vi "Load Settings from XML.vi"(8 "error in (no error)":errorcluster, 11 "Settings in":T1) -> (0 "error out":errorcluster, 3 "Settings out":T1)   [LabVIEW 2022 SP3, in "pm Settings.lvlib"]
doc: "Attempts to load previous user specified settings from an XML file.\n\nThis VI will not generate an error. If a suitable XML file can't be loaded and parsed then it will simply return the default settings."
uses:
  pm Settings.lvlib
  Settings.ctl
  Acquisition/Hardware Configuration.ctl
  Acquisition/Signal Type.ctl
  Logging/Logging Configuration.ctl
  <vilib>/Utility/xml.llb/Read From XML File(string).vi
  <vilib>/Utility/xml.llb/Write to XML File(string).vi
  Acquisition/pm Acquisition.lvlib
  Logging/pm Logging.lvlib
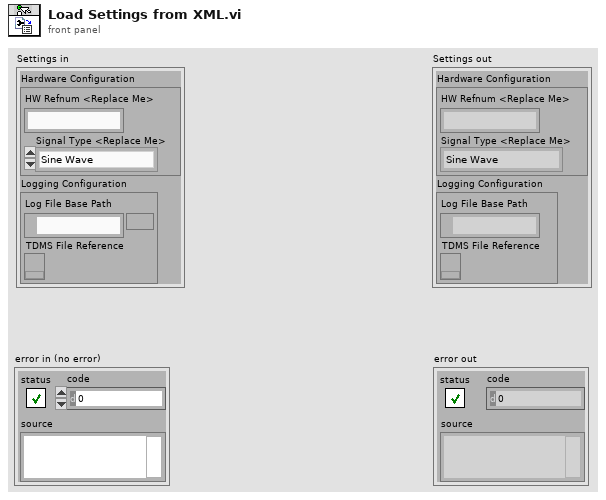
[diagram p1: front panel]
types:
  T1 = typedef "pm Settings.lvlib/Settings.ctl" = cluster{"Hardware Configuration":T2, "Logging Configuration":T4}
  T2 = typedef "pm Acquisition.lvlib/Hardware Configuration.ctl" = cluster{"HW Refnum <Replace Me>":string, "Signal Type <Replace Me>":T3}
  T3 = typedef "pm Acquisition.lvlib/Signal Type.ctl" = enum16{"Sine Wave", "Square with Noise"}
  T4 = typedef "pm Logging.lvlib/Logging Configuration.ctl" = cluster{"Log File Base Path":path, "TDMS File Reference":refnum<k34>}
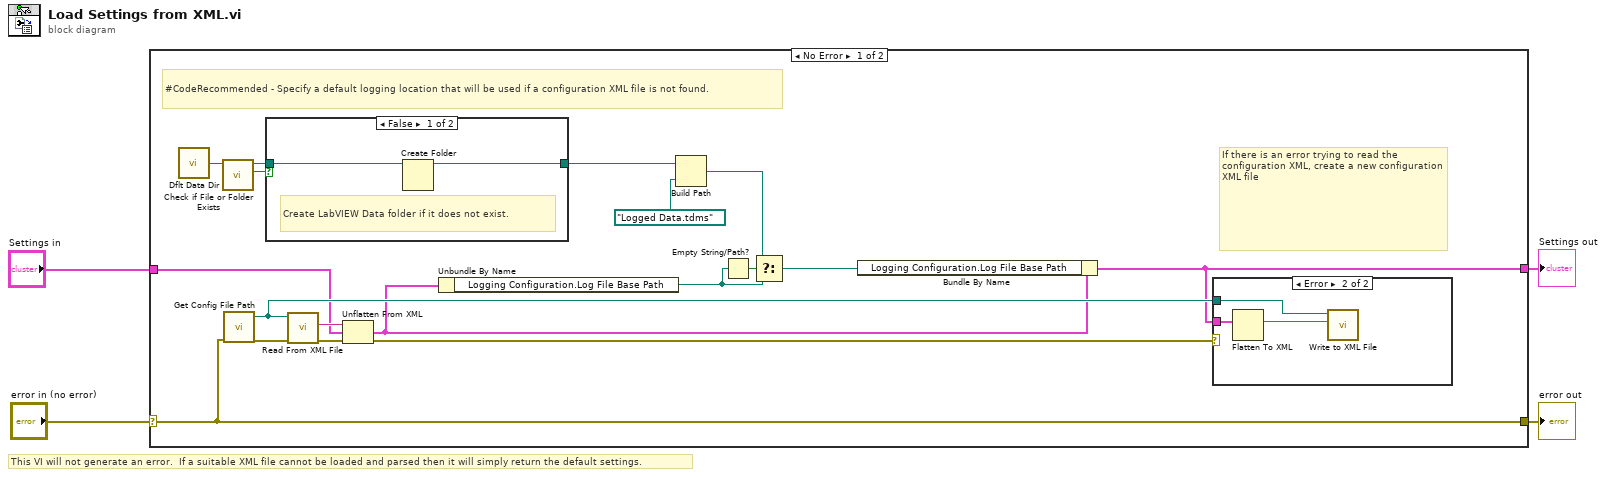
[diagram p0: block diagram]
diagram:
  # "This VI will not generate an error.  If a suitable XML file cannot be loaded and parsed then it will simply return the default settings."
  n1 = case shown="No Error" "error in (no error)" {
    selector: "error in (no error)" -> [w20 w30]
    tunnel: [w20 w30] -> w3
    tunnel: "Settings in" -> [w15 w29]
    tunnel: [w9 w29] -> w1
    frame No Error {
      # "If there is an error trying to read the configuration XML, create a new configuration XML file"
      # "#CodeRecommended - Specify a default logging location that will be used if a configuration XML file is not found."
      n2 = call <vilib>:"Dflt Data Dir.vi"() -> ("App:Default Data Directory"=w8:path)
      n3 = call <vilib>:"Check if File or Folder Exists.vi"("path"=w8) -> ("file or folder exists?"=w7:bool, "dup path"=w6:path)  [unwired: 8 in, 1 out]
      n4 = call "Get Config File Path.vi"("error in (no error)"=w20) -> ("error out"=w22:errorcluster, "XML File Path"=w18:path)  [unwired: 9 in]
      n5 = case shown="False" w7 {
        tunnel: w6 -> [w24 w25]
        tunnel: [w23 w25] -> w5
        frame False {
          # "Create LabVIEW Data folder if it does not exist."
          n6 = Create Folder(path (use dialog)=w24) -> (created path=w23:path)  [unwired: 2 in, 2 out]
        }
        frame True {
        }
      }
      n7 = call-poly <vilib>:"Read From XML File.vi"("error in (no error)"=w22, "XML File Path"=w18) -> ("error out"=w17:errorcluster, "XML Elements"=w21:string)  [unwired: 7 in, 1 out]
      n8 = Unflatten From XML(xml string=w21, type=w15, error in (no error)=w17) -> (value=w11:T1, error out=w16:errorcluster)
      n9 = Unbundle By Name(w11) -> ("Logging Configuration.Log File Base Path"=w13:path)
      n10 = Build Path(base path=w5, name or relative path=path "Logged Data.tdms" ("App:Default Data Directory")) -> (appended path=w12:path)
      n11 = Empty String/Path?(string/path=w13) -> (empty?=w14:bool)
      n12 = Select(t=w12, s=w14, f=w13) -> (s? t:f=w10:path)
      n13 = Bundle By Name(cluster=w11, "Logging Configuration.Log File Base Path"=w10) -> (w9:T1)
      n14 = case shown="Error" w16 {
        tunnel: w9 -> [_ w28]
        tunnel: w18 -> [_ w26]
        frame No Error {
        }
        frame Error {
          n15 = Flatten To XML(6:w28) -> (2:w27:string)
          n16 = call-poly <vilib>:"Write to XML File.vi"("XML Input"=w27, "XML File Path"=w26) -> ()  [unwired: 7 in, 3 out]
        }
      }
    }
    frame Error {
    }
  }
  "error out" <- w3
  "Settings out" <- w1
